vi "Adjust Subs Time.vi"() -> ()   [LabVIEW 2020]
panel:
  in  "Ajuste de tiempo (seg. +/-)":dbl min=-50.0 max=50.0 step=1.0 format="%_2f"
  in  "SRT file in":path
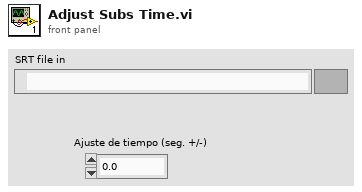
[diagram p1: front panel]
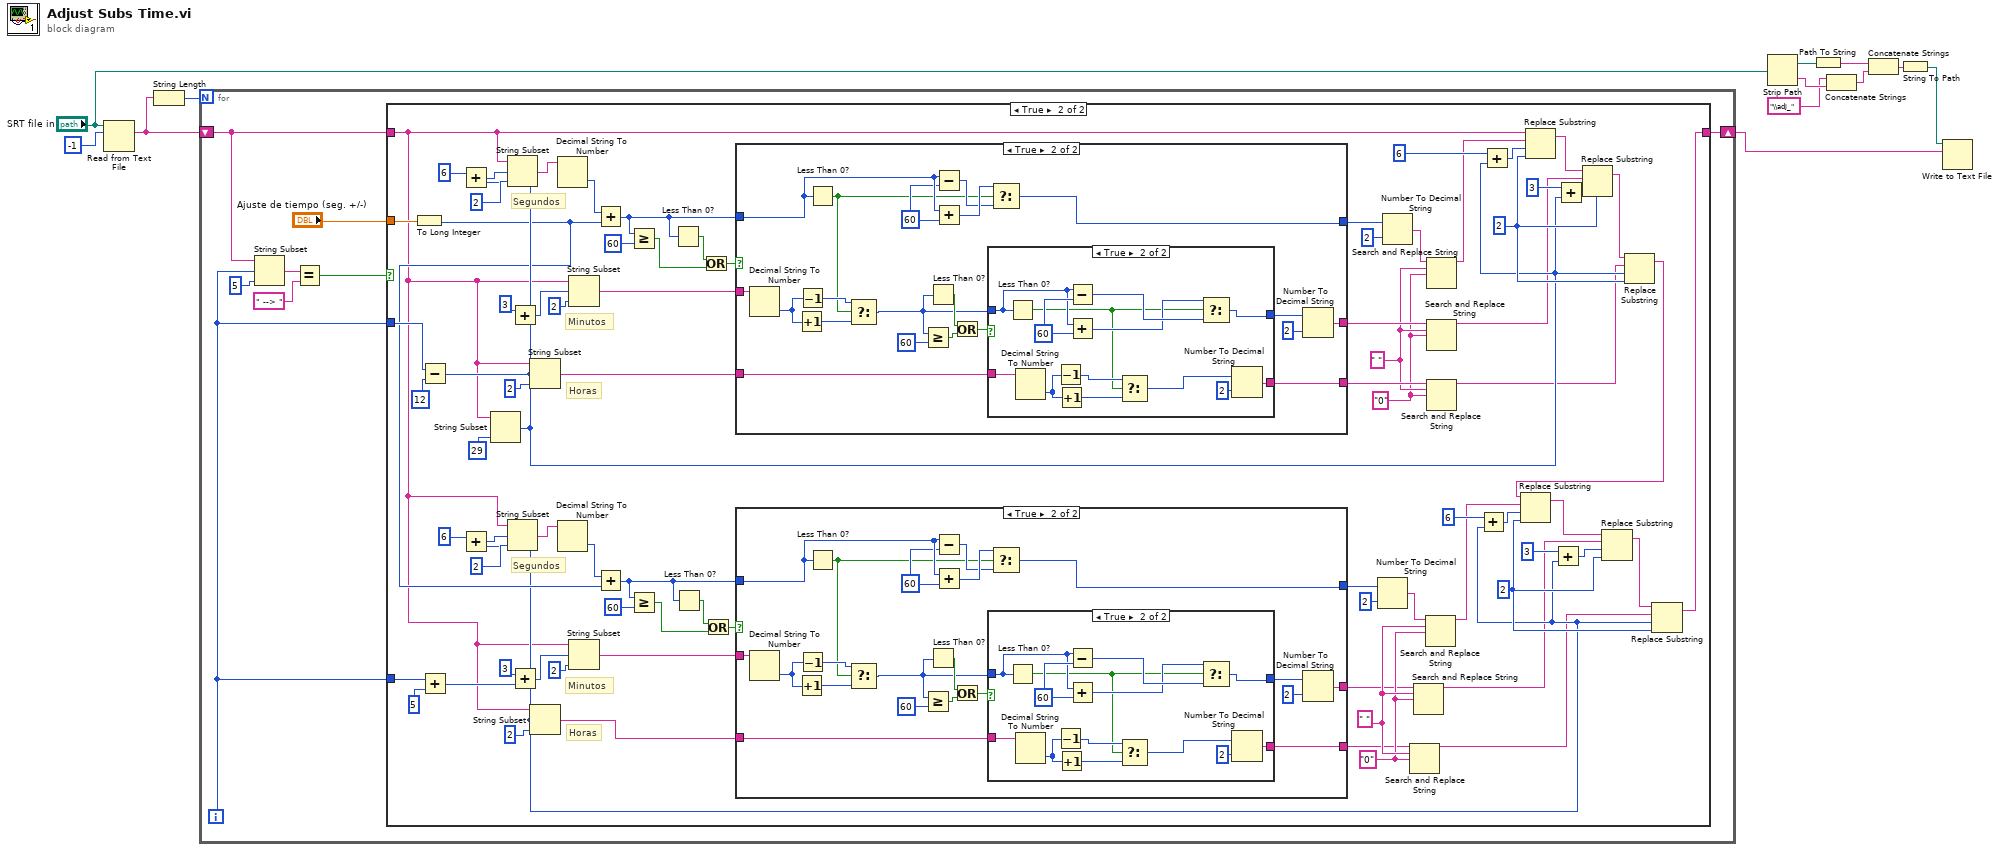
[diagram p0: block diagram]
diagram:
  n1 = Read from Text File(file (use dialog)="SRT file in", count=-1) -> (text=w11:string)  [unwired: 2 in, 3 out]
  n2 = String Length(string=w11) -> (length=w10:i32)
  n3 = for {
    N: w10 -> [_]
    shift-right: [w15] -> w1
    shift-left: w11 -> [w16]
    i -> [w13]
    n4 = String Subset(string=w16, offset (0)=w13, length (rest)=5 ("length (rest)")) -> (substring=w19:string)
    n5 = Equal?(x=w19, y=" --> " ("search string/char (-)")) -> (x = y?=w17:bool)
    n6 = case shown="True" w17 {
      tunnel: w16 -> [w21 w51]
      tunnel: w13 -> [_ w97]
      tunnel: [w21 w57] -> w15
      tunnel: "Ajuste de tiempo (seg. +/-)" -> [_ w91]
      tunnel: w13 -> [_ w55]
      frame False {
      }
      frame True {
        w35 = "0" ("replace string (\"\")")
        w36 = " " ("search string")
        w43 = "0" ("replace string (\"\")")
        w44 = " " ("search string")
        w75 = 2 ("length (len. of substring)")
        w76 = 2 ("length (len. of substring)")
        # "Horas"
        # "Minutos"
        # "Segundos"
        # "Horas"
        # "Minutos"
        # "Segundos"
        n7 = To Long Integer(number=w91) -> (32bit integer=w54:i32)
        n8 = Subtract(x=w97, y=12) -> (x-y=w59:i32)
        n9 = Add(x=w55, y=5) -> (x+y=w52:i32)
        n10 = Add(x=6, y=w59) -> (x+y=w96:i32)
        n11 = Add(x=6, y=w52) -> (x+y=w60:i32)
        n12 = String Subset(string=w51, offset (0)=w59, length (rest)=29 ("length (rest)")) -> ()  [unwired: 1 out]
        n13 = String Subset(string=w51, offset (0)=w96, length (rest)=2 ("length (rest)")) -> (substring=w93:string)
        n14 = String Subset(string=w51, offset (0)=w60, length (rest)=2 ("length (rest)")) -> (substring=w63:string)
        n15 = Add(x=3, y=w59) -> (x+y=w89:i32)
        n16 = Add(x=3, y=w52) -> (x+y=w66:i32)
        n17 = String Subset(string=w51, offset (0)=w59, length (rest)=2 ("length (rest)")) -> (substring=w84:string)
        n18 = String Subset(string=w51, offset (0)=w52, length (rest)=2 ("length (rest)")) -> (substring=w25:string)
        n19 = Decimal String To Number(string=w93) -> (number=w92:i32)  [unwired: 2 in, 1 out]
        n20 = Decimal String To Number(string=w63) -> (number=w64:i32)  [unwired: 2 in, 1 out]
        n21 = String Subset(string=w51, offset (0)=w89, length (rest)=2 ("length (rest)")) -> (substring=w86:string)
        n22 = String Subset(string=w51, offset (0)=w66, length (rest)=2 ("length (rest)")) -> (substring=w26:string)
        n23 = Add(x=w92, y=w54) -> (x+y=w31:i32)
        n24 = Add(x=w64, y=w54) -> (x+y=w27:i32)
        n25 = Greater Or Equal?(x=w31, y=60) -> (x >= y?=w33:bool)
        n26 = Greater Or Equal?(x=w27, y=60) -> (x >= y?=w29:bool)
        n27 = Less Than 0?(x=w31) -> (x < 0?=w32:bool)
        n28 = Less Than 0?(x=w27) -> (x < 0?=w30:bool)
        n29 = Or(x=w32, y=w33) -> (x .or. y?=w34:bool)
        n30 = Or(x=w30, y=w29) -> (x .or. y?=w28:bool)
        n31 = case shown="True" w34 {
          tunnel: w31 -> [w140 w150]
          tunnel: [w140 w148] -> w83
          tunnel: w86 -> [w138 w159]
          tunnel: w84 -> [w139 w157]
          tunnel: [w138 w156] -> w40
          tunnel: [w139 w155] -> w38
          frame False {
          }
          frame True {
            w149 = 60 ("y")
            n32 = Decimal String To Number(string=w159) -> (number=w145:i32)  [unwired: 2 in, 1 out]
            n33 = Increment(x=w145) -> (x+1=w143:i32)
            n34 = Decrement(x=w145) -> (x-1=w144:i32)
            n35 = Less Than 0?(x=w150) -> (x < 0?=w142:bool)
            n36 = Select(t=w144, s=w142, f=w143) -> (s? t:f=w141:i32)
            n37 = Greater Or Equal?(x=w141, y=60) -> (x >= y?=w151:bool)
            n38 = Less Than 0?(x=w141) -> (x < 0?=w153:bool)
            n39 = Subtract(x=w150, y=w149) -> (x-y=w146:i32)
            n40 = Add(x=w150, y=w149) -> (x+y=w147:i32)
            n41 = Or(x=w153, y=w151) -> (x .or. y?=w152:bool)
            n42 = case shown="True" w152 {
              tunnel: w141 -> [w162 w171]
              tunnel: [w162 w163] -> w158
              tunnel: w157 -> [w161 w175]
              tunnel: [w161 w174] -> w155
              frame False {
              }
              frame True {
                w172 = 60 ("y")
                n43 = Less Than 0?(x=w171) -> (x < 0?=w165:bool)
                n44 = Decimal String To Number(string=w175) -> (number=w168:i32)  [unwired: 2 in, 1 out]
                n45 = Decrement(x=w168) -> (x-1=w166:i32)
                n46 = Increment(x=w168) -> (x+1=w167:i32)
                n47 = Subtract(x=w171, y=w172) -> (x-y=w170:i32)
                n48 = Add(x=w171, y=w172) -> (x+y=w169:i32)
                n49 = Select(t=w166, s=w165, f=w167) -> (s? t:f=w164:i32)
                n50 = Select(t=w169, s=w165, f=w170) -> (s? t:f=w163:i32)
                n51 = Number To Decimal String(number=w164, width (-)=i16 2) -> (decimal integer string=w174:string)
              }
            }
            n52 = Select(t=w147, s=w142, f=w146) -> (s? t:f=w148:i32)
            n53 = Number To Decimal String(number=w158, width (-)=i16 2) -> (decimal integer string=w156:string)
          }
        }
        n54 = case shown="True" w28 {
          tunnel: w27 -> [w102 w112]
          tunnel: [w102 w110] -> w24
          tunnel: w26 -> [w100 w121]
          tunnel: w25 -> [w101 w119]
          tunnel: [w100 w118] -> w23
          tunnel: [w101 w117] -> w22
          frame False {
          }
          frame True {
            w111 = 60 ("y")
            n55 = Decimal String To Number(string=w121) -> (number=w107:i32)  [unwired: 2 in, 1 out]
            n56 = Increment(x=w107) -> (x+1=w105:i32)
            n57 = Decrement(x=w107) -> (x-1=w106:i32)
            n58 = Less Than 0?(x=w112) -> (x < 0?=w104:bool)
            n59 = Select(t=w106, s=w104, f=w105) -> (s? t:f=w103:i32)
            n60 = Greater Or Equal?(x=w103, y=60) -> (x >= y?=w113:bool)
            n61 = Less Than 0?(x=w103) -> (x < 0?=w115:bool)
            n62 = Subtract(x=w112, y=w111) -> (x-y=w108:i32)
            n63 = Add(x=w112, y=w111) -> (x+y=w109:i32)
            n64 = Or(x=w115, y=w113) -> (x .or. y?=w114:bool)
            n65 = case shown="True" w114 {
              tunnel: w103 -> [w124 w133]
              tunnel: [w124 w125] -> w120
              tunnel: w119 -> [w123 w137]
              tunnel: [w123 w136] -> w117
              frame False {
              }
              frame True {
                w134 = 60 ("y")
                n66 = Less Than 0?(x=w133) -> (x < 0?=w127:bool)
                n67 = Decimal String To Number(string=w137) -> (number=w130:i32)  [unwired: 2 in, 1 out]
                n68 = Decrement(x=w130) -> (x-1=w128:i32)
                n69 = Increment(x=w130) -> (x+1=w129:i32)
                n70 = Subtract(x=w133, y=w134) -> (x-y=w132:i32)
                n71 = Add(x=w133, y=w134) -> (x+y=w131:i32)
                n72 = Select(t=w128, s=w127, f=w129) -> (s? t:f=w126:i32)
                n73 = Select(t=w131, s=w127, f=w132) -> (s? t:f=w125:i32)
                n74 = Number To Decimal String(number=w126, width (-)=i16 2) -> (decimal integer string=w136:string)
              }
            }
            n75 = Select(t=w109, s=w104, f=w108) -> (s? t:f=w110:i32)
            n76 = Number To Decimal String(number=w120, width (-)=i16 2) -> (decimal integer string=w118:string)
          }
        }
        n77 = Number To Decimal String(number=w24, width (-)=i16 2) -> (decimal integer string=w45:string)
        n78 = Number To Decimal String(number=w83, width (-)=i16 2) -> (decimal integer string=w42:string)
        n79 = Search and Replace String(input string=w22, search string=w44, replace string=w43) -> (result string=w48:string)  [unwired: 5 in, 3 out]
        n80 = Search and Replace String(input string=w23, search string=w44, replace string=w43) -> (result string=w47:string)  [unwired: 5 in, 3 out]
        n81 = Search and Replace String(input string=w45, search string=w44, replace string=w43) -> (result string=w46:string)  [unwired: 5 in, 3 out]
        n82 = Search and Replace String(input string=w42, search string=w36, replace string=w35) -> (result string=w41:string)  [unwired: 5 in, 3 out]
        n83 = Search and Replace String(input string=w40, search string=w36, replace string=w35) -> (result string=w39:string)  [unwired: 5 in, 3 out]
        n84 = Search and Replace String(input string=w38, search string=w36, replace string=w35) -> (result string=w37:string)  [unwired: 5 in, 3 out]
        n85 = Add(x=6, y=w52) -> (x+y=w74:i32)
        n86 = Add(x=6, y=w59) -> (x+y=w77:i32)
        n87 = Replace Substring(2:w76, 3:w77, 4:w41, 5:w51) -> (1:w82:string)  [unwired: 1 out]
        n88 = Add(x=3, y=w52) -> (x+y=w71:i32)
        n89 = Add(x=3, y=w59) -> (x+y=w80:i32)
        n90 = Replace Substring(2:w76, 3:w80, 4:w39, 5:w82) -> (1:w81:string)  [unwired: 1 out]
        n91 = Replace Substring(2:w76, 3:w59, 4:w37, 5:w81) -> (1:w58:string)  [unwired: 1 out]
        n92 = Replace Substring(2:w75, 3:w74, 4:w46, 5:w58) -> (1:w69:string)  [unwired: 1 out]
        n93 = Replace Substring(2:w75, 3:w71, 4:w47, 5:w69) -> (1:w70:string)  [unwired: 1 out]
        n94 = Replace Substring(2:w75, 3:w52, 4:w48, 5:w70) -> (1:w57:string)  [unwired: 1 out]
      }
    }
  }
  n95 = Strip Path(path="SRT file in") -> (stripped path=w9:path, name=w4:string)
  n96 = Path To String(path=w9) -> (string=w8:string)
  n97 = Concatenate Strings("\\adj_" ("string"), w4) -> (w5:string)
  n98 = Concatenate Strings(w8, w5) -> (w7:string)
  n99 = String To Path(string=w7) -> (path=w2:path)
  n100 = Write to Text File(file (use dialog)=w2, text=w1) -> ()  [unwired: 2 in, 3 out]
